vi "Open or Close front panel of caller.vi"(4 "Error Processing":enum16{"Active Errors", "Inactive Errors"}(ring)=enum."Inactive Errors", 5 "Control":enum16{"Open", "Close", "Status", "No Change"}(ring), 6 "error in (no error)":errorcluster, 8 "VI Refnum in":refnum<vi>, 9 "Is Dialog?":enum16{"Normal", "Dialog Box"}(ring)) -> (0 "error out":errorcluster, 1 "Dialog Box?":bool, 2 "Calling VI":string, 3 "Panel Open?":bool, 7 "VI Refnum out":refnum<vi>)   [LabVIEW 2013]
doc: "This VI will allow the front panel of the calling VI to be programatically opened or closed, or the status of the panel may be querried. Also this vi may be used to set or revoke the dialog box attribute of the front panel. If not wired, the dialog box attribute defaults to normal window operation (not dialog box)."
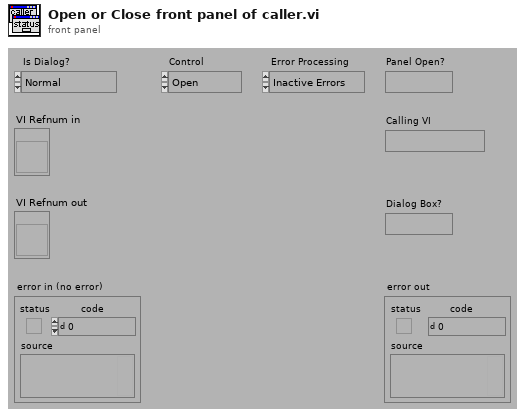
[diagram p1: front panel]
types:
  T1 = enum32{"Invalid", "Standard", "Closed", "Hidden", "Minimized", "Maximized"}
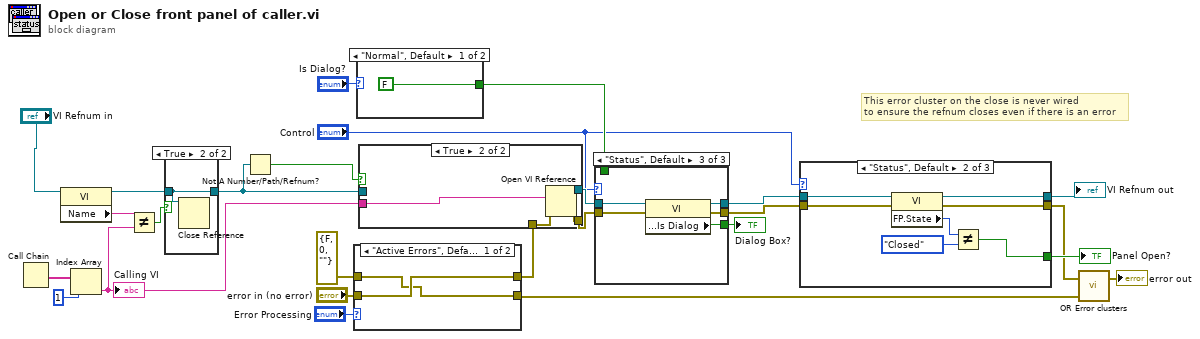
[diagram p0: block diagram]
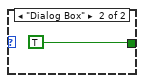
[diagram p4: hidden frame]
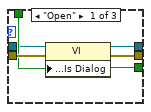
[diagram p5: hidden frame]
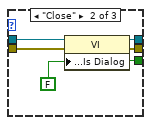
[diagram p6: hidden frame]
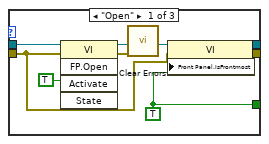
[diagram p8: hidden frame]
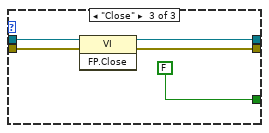
[diagram p9: hidden frame]
diagram:
  # "This error cluster on the close is never wired\nto ensure the refnum closes even if there is an error"
  n1 = Call Chain() -> (call chain=w6:string[])
  n2 = property class="VI"(reference="VI Refnum in") -> (reference out=w3:refnum<vi>, "Name"=w5:string)  [unwired: 1 in, 1 out]
  n3 = Index Array(array=w6, index=1) -> (element=w1:string)
  "Calling VI" <- w1
  n4 = Not Equal?(x=w5, y=w1) -> (x != y?=w4:bool)
  n5 = case shown="True" w4 {
    tunnel: w3 -> [w27 w28]
    tunnel: [w27 w28] -> w2
    frame False {
    }
    frame True {
      n6 = Close Reference(reference=w28) -> ()  [unwired: 1 in, 1 out]
    }
  }
  n7 = Not A Number/Path/Refnum?(number/path/refnum=w2) -> (NaN/Path/Refnum?=w9:bool)
  n8 = case shown="\"Active Errors\", Default" "Error Processing" {
    tunnel: "error in (no error)" -> [w30 w32]
    tunnel: [w30 w31] -> w10
    tunnel: [w29 w32] -> w21
    tunnel: errorcluster {"status"=FALSE, "code"=0, "source"=""} ("error in (no error)") -> [w29 w31]
    frame "Active Errors", Default {
    }
    frame "Inactive Errors" {
    }
  }
  n9 = case shown="\"Normal\", Default" "Is Dialog?" {
    tunnel: [FALSE TRUE] -> w18
    frame "Normal", Default {
    }
    frame "Dialog Box" {
    }
  }
  n10 = case shown="True" w9 {
    tunnel: [w35 w40] -> w16
    tunnel: [w36 w39] -> w15
    tunnel: w10 -> [w36 w38]
    tunnel: w2 -> [w35 _]
    tunnel: w1 -> [_ w37]
    frame False {
    }
    frame True {
      n11 = Open VI Reference(vi path=w37, error in (no error)=w38) -> (vi reference=w40:refnum<vi>, error out=w39:errorcluster)  [unwired: 1 in, 3 out]
    }
  }
  n12 = case shown="\"Status\", Default" "Control" {
    tunnel: w16 -> [w41 w48 w55]
    tunnel: [w45 w50 w54] -> w14
    tunnel: w15 -> [w44 w47 w52]
    tunnel: [w43 w49 w53] -> w13
    tunnel: [w42 w46 w51] -> w20
    tunnel: w18 -> [w42 _ _]
    frame "Open" {
      n13 = property class="VI"(reference=w41, error in=w44, "Front Panel Window:Is Dialog"=w42) -> (reference out=w45:refnum<vi>, error out=w43:errorcluster)
    }
    frame "Close" {
      w46 = FALSE ("Front Panel Window:Is Dialog")
      n14 = property class="VI"(reference=w48, error in=w47, "Front Panel Window:Is Dialog"=w46) -> (reference out=w50:refnum<vi>, error out=w49:errorcluster)
    }
    frame "Status", Default {
      n15 = property class="VI"(reference=w55, error in=w52) -> (reference out=w54:refnum<vi>, error out=w53:errorcluster, "Front Panel Window:Is Dialog"=w51:bool)
    }
  }
  "Dialog Box?" <- w20
  n16 = case shown="\"Status\", Default" "Control" {
    tunnel: w14 -> [w59 w67 w73]
    tunnel: [w63 w70 w72] -> w12
    tunnel: w13 -> [w56 w68 w74]
    tunnel: [w61 w64 FALSE ("Front Panel.Open")] -> w26
    tunnel: [w62 w69 w71] -> w17
    frame "Open" {
      w61 = TRUE ("Front Panel.Open")
      n17 = invoke class="VI" method="FP.Open"(reference=w59, error in=w56, "Activate"=TRUE ("Activate?")) -> (reference out=w58:refnum<vi>, error out=w60:errorcluster)  [unwired: 2 in, 3 out]
      n18 = call <vilib>:"Clear Errors.vi"("error in (no error)"=w60) -> ()  [unwired: 6 in, 1 out]
      n19 = property class="VI"(reference=w58, error in=w56, "Front Panel.IsFrontmost"=w61) -> (reference out=w62:refnum<vi>, error out=w63:errorcluster)
    }
    frame "Status", Default {
      n20 = property class="VI"(reference=w67, error in=w68) -> (reference out=w69:refnum<vi>, error out=w70:errorcluster, "FP.State"=w66:T1)
      n21 = Not Equal?(x=w66, y=T1."Closed") -> (x != y?=w64:bool)
    }
    frame "Close" {
      n22 = invoke class="VI" method="FP.Close"(reference=w73, error in=w74) -> (reference out=w71:refnum<vi>, error out=w72:errorcluster)  [unwired: 1 in, 1 out]
    }
  }
  "Panel Open?" <- w26
  "VI Refnum out" <- w17
  n23 = call "OR Error clusters.vi"("error in 2"=w21, "error in 1"=w12) -> ("error out"=→"error out":errorcluster)  [unwired: 1 out]
